vi "Vision Processing Backup 31 Jan.vi"() -> ()   [LabVIEW 2016]
uses:
  <vilib>/Rock Robotics/WPI/Camera/WPI_CameraImageSize.ctl
  <vilib>/Rock Robotics/WPI/Camera/WPI_CameraWhite Balance Values.ctl
  <vilib>/Rock Robotics/WPI/Camera/WPI_CameraExposure Values.ctl
  <vilib>/Rock Robotics/WPI/Camera/WPI_CameraFrameRate.ctl
  Robot Global Data.vi
  <vilib>/vision/NI_Vision_Development_Module.lvlib
panel:
  in  "Image Size":T1=enum."320x240"
  in  "error in (no error)":errorcluster
  out "Image":T2(plugin-control)
  out "error out":errorcluster
  out "Image 2":T2(plugin-control)
  in  "Range":cluster{"Lower value":sgl, "Upper value":sgl}={"Lower value"=128.0, "Upper value"=255.0}
  in  "Color Plane":i32(ring)=7 items=["Red", "Green", "Blue", "Hue", "Saturation", "Luminance", "Value", "Intensity"]
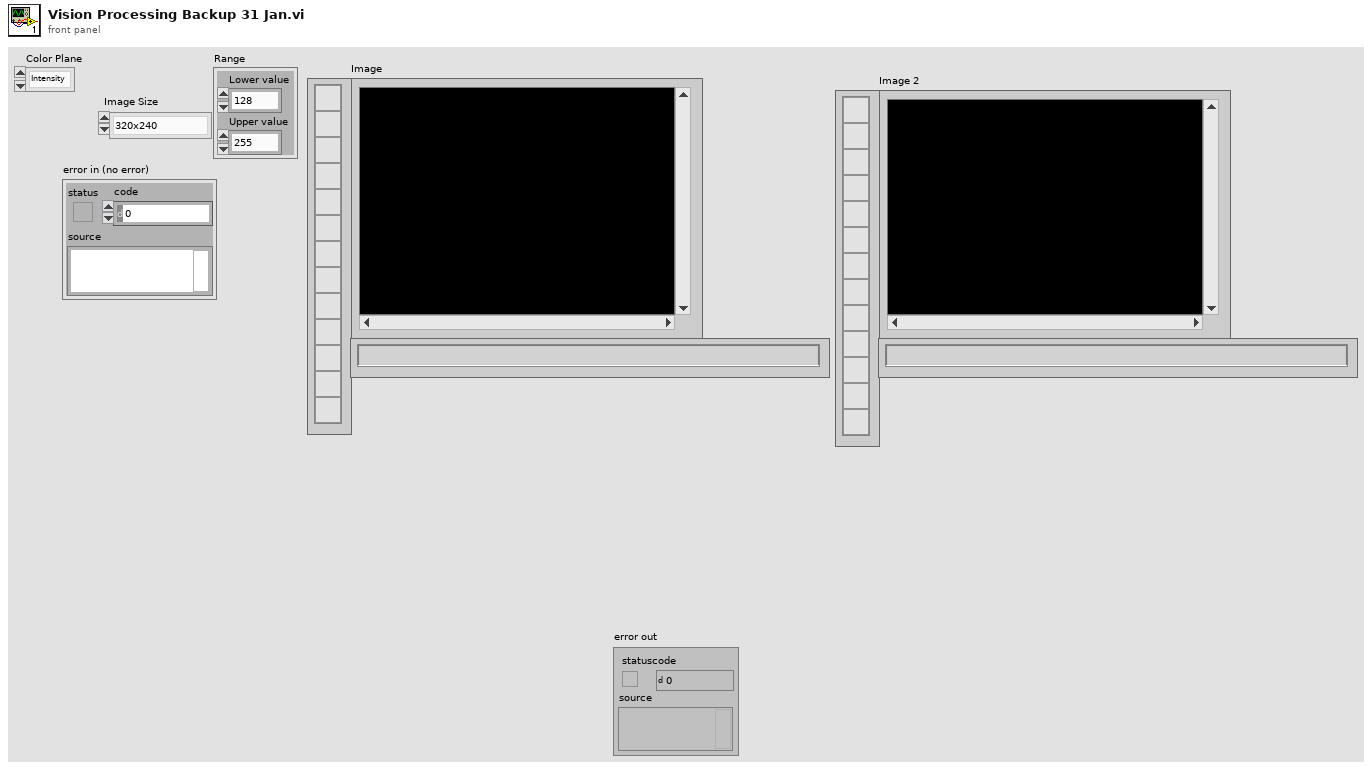
[diagram p1: front panel]
types:
  T1 = typedef "WPI_CameraImageSize.ctl" = enum16{"640x480", "320x240", "160x120", "Custom"}
  T2 = typedef "IMAQ Image.ctl" = refnum<image>
  T3 = typedef "Image Type" = u32
  T4 = typedef "WPI_CameraFrameRate.ctl" = u32
  T5 = typedef "WPI_CameraExposure Values.ctl" = enum16{"Auto", "Flicker-free 50 Hz", "Flicker-free 60 Hz", "Hold current", "Custom"}
  T6 = typedef "WPI_CameraWhite Balance Values.ctl" = enum16{"Auto", "Fixed indoor", "Fixed outdoor 1", "Fixed outdoor 2", "Fixed fluorescent 1", "Fixed fluorescent 2", "Hold current", "Custom"}
  T7 = typedef "WPI_CameraDevRef.ctl" = cluster{"Camera Address":string, "CameraStatus":errorcluster}
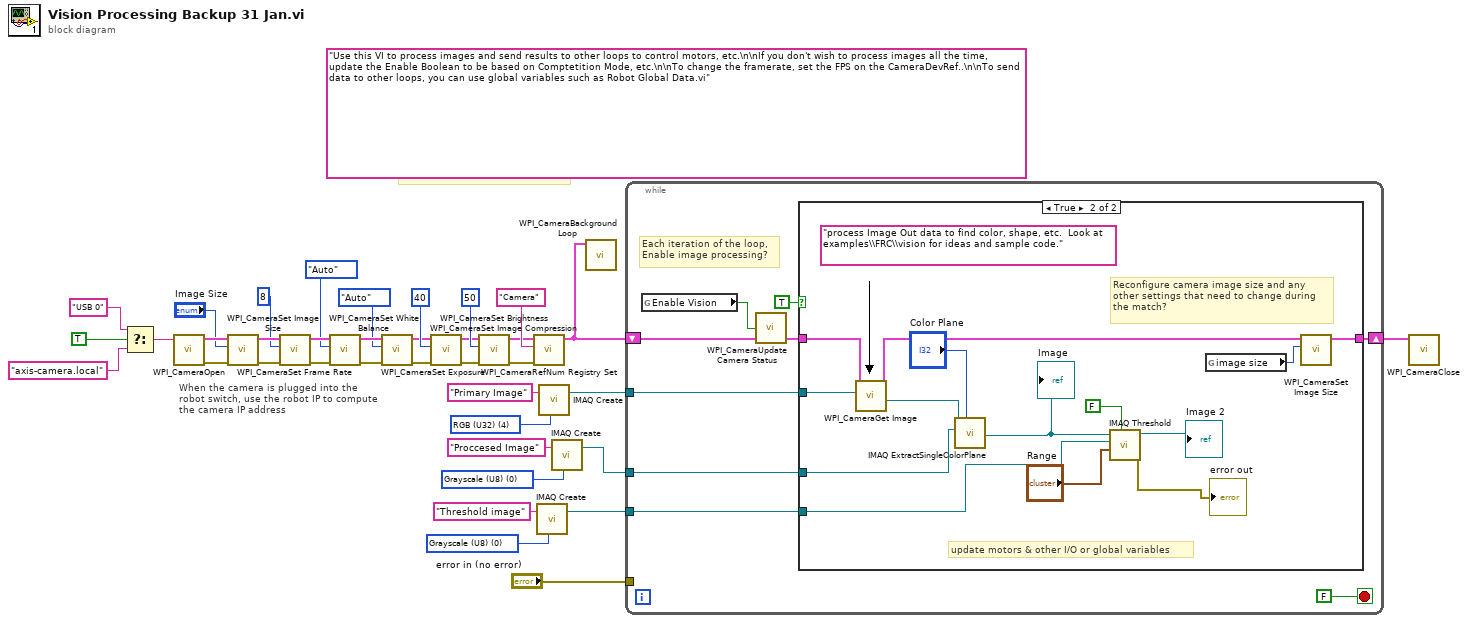
[diagram p0: block diagram]
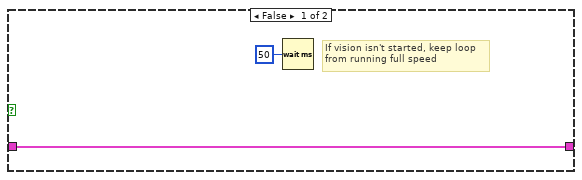
[diagram p2: hidden frame]
diagram:
  w2 = T3 0 items=["Grayscale (U8)", "Grayscale (I16)", "Grayscale (SGL)", "Complex (CSG)", "RGB (U32)", "HSL (U32)", "RGB (U64)"] ("Image Type")
  w5 = T3 0 items=["Grayscale (U8)", "Grayscale (I16)", "Grayscale (SGL)", "Complex (CSG)", "RGB (U32)", "HSL (U32)", "RGB (U64)"] ("Image Type")
  (unwired) "Use this VI to process images and send results to other loops to control motors, etc.\n\nIf you don't wish to process images all the time, update the Enable Boolean to be based on Comptetition Mode, etc.\n\nTo change the framerate, set the FPS on the CameraDevRef..\n\nTo send data to other loops, you can use global variables such as Robot Global Data.vi"
  w37 = T3 4 items=["Grayscale (U8)", "Grayscale (I16)", "Grayscale (SGL)", "Complex (CSG)", "RGB (U32)", "HSL (U32)", "RGB (U64)"] ("Image Type")
  # "When the camera is plugged into the\nrobot switch, use the robot IP to compute\nthe camera IP address"
  # "For Axis cameras, this reads\nimages continuously to avoid\nlatency. For USB, it optionally\nforwards compressed images to\nthe dashboard process."
  n1 = Select(t="USB 0" ("format string"), s=TRUE ("dot notation? (F)"), f="axis-camera.local" ("format string")) -> (s? t:f=w8:string)
  n2 = call <vilib>:"WPI_CameraOpen.vi"("Camera Address"=w8) -> ("error out"=w25:errorcluster, "CameraDevRef"=w26:T7)  [unwired: 1 in, 8 out]
  n3 = call <vilib>:"WPI_CameraSet Image Size.vi"("error in (no error)"=w25, "Image Size"="Image Size", "CameraDevRef"=w26) -> ("error out"=w24:errorcluster, "CameraDevRef Out"=w27:T7)  [unwired: 1 in, 6 out]
  n4 = call <vilib>:"WPI_CameraSet Frame Rate.vi"("error in (no error)"=w24, "Frame Rate (fps)"=T4 8, "CameraDevRef"=w27) -> ("error out"=w23:errorcluster, "CameraDevRef Out"=w29:T7)  [unwired: 7 out]
  n5 = call <vilib>:"WPI_CameraSet White Balance.vi"("error in (no error)"=w23, "White Balance"=WPI_CameraWhite_Balance_Values."Auto", "CameraDevRef"=w29) -> ("error out"=w22:errorcluster, "CameraDevRef Out"=w28:T7)  [unwired: 1 in, 6 out]
  n6 = call <vilib>:"WPI_CameraSet Exposure.vi"("error in (no error)"=w22, "Exposure"=WPI_CameraExposure_Values."Auto", "CameraDevRef"=w28) -> ("error out"=w21:errorcluster, "CameraDevRef Out"=w31:T7)  [unwired: 1 in, 6 out]
  n7 = call <vilib>:"WPI_CameraSet Image Compression.vi"("error in (no error)"=w21, "Compression"=40, "CameraDevRef"=w31) -> ("error out"=w20:errorcluster, "CameraDevRef Out"=w30:T7)  [unwired: 7 out]
  n8 = call <vilib>:"WPI_CameraSet Brightness.vi"("error in (no error)"=w20, "Brightness"=50, "CameraDevRef"=w30) -> ("error out"=w18:errorcluster, "CameraDevRef Out"=w19:T7)  [unwired: 7 out]
  n9 = call <vilib>:"WPI_CameraRefNum Registry Set.vi"("error in (no error)"=w18, "refnum name"="Camera", "CameraDevRef"=w19) -> ("CameraDevRef"=w14:T7)  [unwired: 1 in, 7 out]
  n10 = call "IMAQ Create"("Image Name"="Threshold image", "Image Type"=w2) -> ("New Image"=w1:T2)  [unwired: 2 in, 2 out]
  n11 = call "IMAQ Create"("Image Name"="Primary Image", "Image Type"=w37) -> ("New Image"=w35:T2)  [unwired: 2 in, 2 out]
  n12 = call "IMAQ Create"("Image Name"="Proccesed Image", "Image Type"=w5) -> ("New Image"=w4:T2)  [unwired: 2 in, 2 out]
  n13 = call <vilib>:"WPI_CameraBackground Loop.vi"("CameraDevRef"=w14) -> ()  [unwired: 11 in]
  n14 = while {
    shift-right: [w45] -> w12
    shift-left: w14 -> [w43]
    tunnel: w35 -> [w44]
    tunnel: "error in (no error)" -> [_]
    tunnel: w4 -> [w40]
    tunnel: w1 -> [w38]
    stop <- FALSE stop-if-true
    # "Each iteration of the loop,\nEnable image processing?"
    n15 = global read "Robot Global Data.vi" "Enable Vision"() -> (w41:bool)
    n16 = call <vilib>:"WPI_CameraUpdate Camera Status.vi"("CameraDevRef In"=w43, "Enable Vision"=w41) -> ("CameraDevRef Out"=w42:T7)  [unwired: 3 in]
    n17 = case shown="True" TRUE {
      tunnel: w44 -> [_ w61]
      tunnel: [w48 w62] -> w45
      tunnel: w42 -> [w48 w59]
      tunnel: w40 -> [_ w56]
      tunnel: w38 -> [_ w53]
      frame False {
        # "If vision isn't started, keep loop\nfrom running full speed"
        n18 = Wait (ms)(milliseconds to wait=u32 50) -> ()  [unwired: 1 out]
      }
      frame True {
        (unwired) "process Image Out data to find color, shape, etc.  Look at examples\\FRC\\vision for ideas and sample code."
        # "update motors & other I/O or global variables"
        # "Reconfigure camera image size and any\nother settings that need to change during\nthe match?"
        n19 = call <vilib>:"WPI_CameraGet Image.vi"("Image"=w61, "CameraDevRef"=w59) -> ("Image Out"=w57:T2, "CameraDevRef Out"=w58:T7)  [unwired: 1 in, 7 out]
        n20 = call "IMAQ ExtractSingleColorPlane"("Color Plane"="Color Plane", "Image Dst"=w56, "Image Src"=w57) -> ("Image Dst Out"=w54:T2)  [unwired: 7 in, 1 out]
        "Image" <- w54
        n21 = call "IMAQ Threshold"("Keep/Replace Value (Replace)"=FALSE, "Range"="Range", "Image Dst"=w53, "Image Src"=w54) -> ("error out"=→"error out":errorcluster, "Image Dst Out"=→"Image 2":T2)  [unwired: 6 in]
        n22 = global read "Robot Global Data.vi" "image size"() -> (w60:T1)
        n23 = call <vilib>:"WPI_CameraSet Image Size.vi"("Image Size"=w60, "CameraDevRef"=w58) -> ("CameraDevRef Out"=w62:T7)  [unwired: 2 in, 7 out]
      }
    }
  }
  n24 = call <vilib>:"WPI_CameraClose.vi"("CameraDevRef"=w12) -> ()  [unwired: 1 in, 10 out]
